vi "Create Laser Controller.vi"(8 "error in (no error)":errorcluster, 10 "Laser Driver.lvclass":refnum<class "Laser Driver.lvclass">) -> (0 "error out":errorcluster, 3 "Laser Controller out":refnum<class "Laser Controller.lvclass">)   [LabVIEW 2022 SP3, in "Laser Controller.lvclass"]
uses:
  Laser Controller.lvclass
  Laser Controller.lvclass/Laser Controller.ctl
  Laser Process/Laser Process/Laser Process.lvclass
  Laser Driver/Laser Driver.lvclass
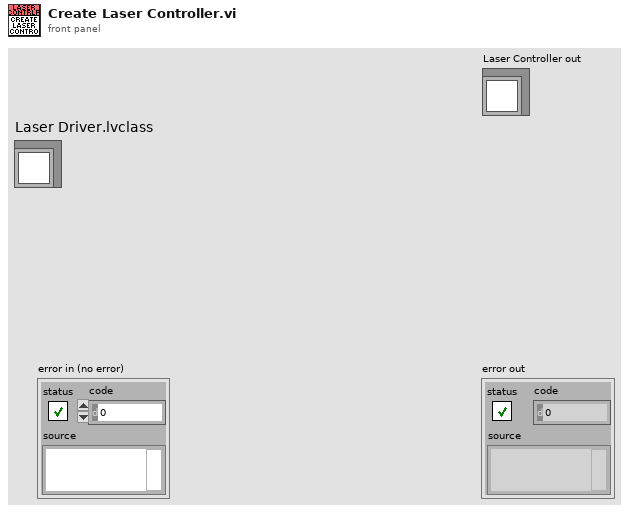
[diagram p1: front panel]
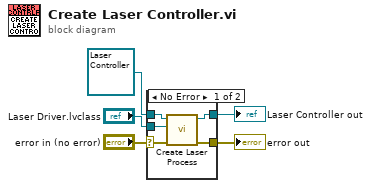
[diagram p0: block diagram]
diagram:
  n1 = case shown="No Error" "error in (no error)" {
    selector: "error in (no error)" -> [w7 w12]
    tunnel: [w6 w12] -> w4
    tunnel: [w8 w11] -> w3
    tunnel: refnum<class "Laser Controller.lvclass"> refnum ("Laser Controller in") -> [w9 w11]
    tunnel: "Laser Driver.lvclass" -> [w10 _]
    frame No Error {
      n2 = call "Create Laser Process.vi"("error in (no error)"=w7, "Laser Driver.lvclass"=w10, "Laser Controller in"=w9) -> ("error out"=w6:errorcluster, "Laser Controller"=w8:refnum<class "Laser Controller.lvclass">)  [unwired: 7 in]
    }
    frame Error {
    }
  }
  "error out" <- w4
  "Laser Controller out" <- w3
